vi "Execute.vi"(8 "error in (no error)":errorcluster, 10 "Abstract Consumer in":refnum<class "Abstract Consumer.lvclass">, 11 "Switch Connect Message in":refnum<class "Switch Connect Message.lvclass">) -> (0 "error out":errorcluster, 1 "Abstract Response out":refnum<class "Abstract Response Message.lvclass">, 2 "Abstract Consumer out":refnum<class "Abstract Consumer.lvclass">, 3 "Switch Connect Message out":refnum<class "Switch Connect Message.lvclass">, 4 "Stop?":bool)   [LabVIEW 2017, in "Messaging.lvlib" / "Switch Connect Message.lvclass"]
uses:
  Switch Connect Message.lvclass
  Consumer/Abstract Consumer/Abstract Consumer.lvclass
  Message/Abstract Response Message/Abstract Response Message.lvclass
  Abstract Switch Consumer/Abstract Switch Consumer.lvclass
  C:/github/niveristand-custom-device-message-library/Source/Consumer/Abstract Consumer/Abstract Consumer.lvclass
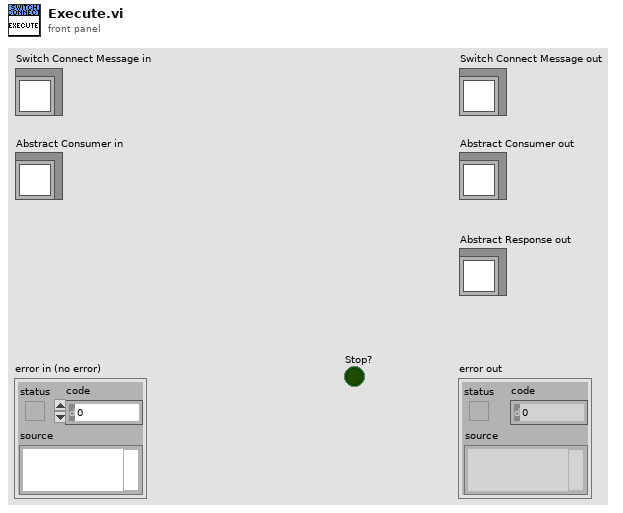
[diagram p1: front panel]
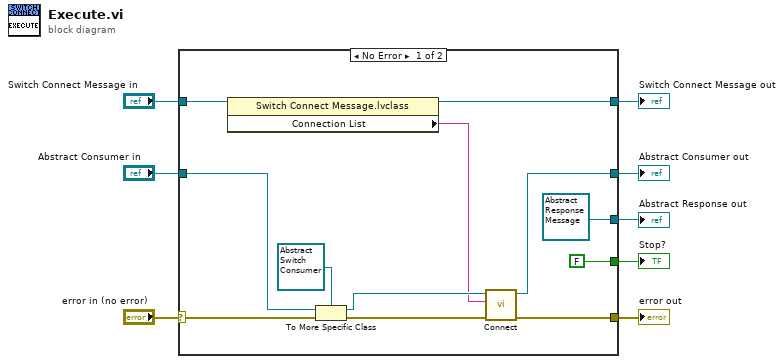
[diagram p0: block diagram]
diagram:
  n1 = case shown="No Error" "error in (no error)" {
    selector: "error in (no error)" -> [w19 w23]
    tunnel: [w15 w23] -> w7
    tunnel: [w11 w22] -> w6
    tunnel: "Switch Connect Message in" -> [w12 w22]
    tunnel: "Abstract Consumer in" -> [w20 w21]
    tunnel: [w14 w21] -> w3
    tunnel: [FALSE ("Stop?") _] -> w2
    tunnel: [refnum<class "Abstract Response Message.lvclass"> refnum ("Abstract Response out") _] -> w1
    frame No Error {
      n2 = property class="Switch Connect Message.lvclass"(reference=w12) -> (reference out=w11:refnum<class "Switch Connect Message.lvclass">, "Connection List"=w13:string)  [unwired: 1 in, 1 out]
      n3 = To More Specific Class(target class=refnum<class "Abstract Switch Consumer.lvclass"> refnum ("Message Queue Library.lvlib:Abstract Switch Consumer.lvclass"), reference=w20, error in=w19) -> (specific class reference=w16:refnum<class "Abstract Switch Consumer.lvclass">, error out=w17:errorcluster)
      n4 = call-dynamic "Connect.vi"("error in (no error)"=w17, "Connection list in"=w13, "Abstract Switch Consumer in"=w16) -> ("error out"=w15:errorcluster, "Abstract Switch Consumer out"=w14:refnum<class "Abstract Switch Consumer.lvclass">)  [unwired: 7 in]
    }
    frame Error {
    }
  }
  "error out" <- w7
  "Switch Connect Message out" <- w6
  "Abstract Consumer out" <- w3
  "Stop?" <- w2
  "Abstract Response out" <- w1
